vi "Lang Set Desc b.vi"(8 "error in (no error)":errorcluster, 10 "b":T1, 11 "LF2R IDE in":refnum<class "Main Panel.lvclass">) -> (0 "error out":errorcluster, 3 "LF2R IDE out":refnum<class "Main Panel.lvclass">)   [LabVIEW 2018, in "Framework.lvlib" / "Framework.lvclass"]
uses:
  Framework/Framework/Framework.lvclass
  Main Panel.lvclass
  D:/project/hobby/LabVIEW/LF2R/LabVIEW/Source/Actor/Framework/Framework/Framework.lvclass
  C:/Program Files (x86)/National Instruments/LabVIEW 2018/vi.lib/MGI/Panel Manager/Panel Actor/Panel Actor/Panel Actor.lvclass
  C:/Program Files (x86)/National Instruments/LabVIEW 2018/vi.lib/MGI/Monitored Actor/Monitored Actor/Monitored Actor/Monitored Actor.lvclass
  C:/Program Files (x86)/National Instruments/LabVIEW 2018/vi.lib/ActorFramework/Actor/Actor.lvclass
  Const Lang Property.ctl
  Const UI Desc Frame b.ctl
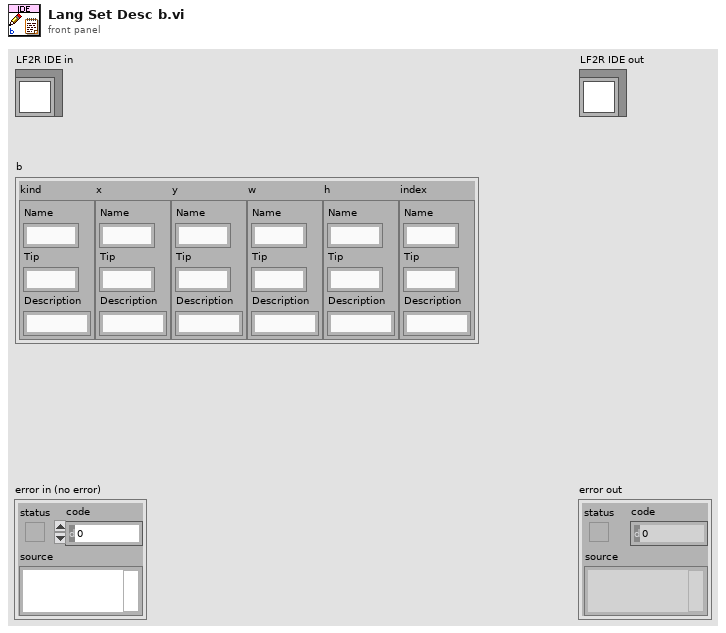
[diagram p1: front panel]
types:
  T1 = typedef "Framework.lvlib/Framework.lvclass/Const UI Desc Frame b.ctl" = cluster{"kind":T2, "x":T2, "y":T2, "w":T2, "h":T2, "index":T2}
  T2 = typedef "Framework.lvlib/Framework.lvclass/Const Lang Property.ctl" = cluster{"Name":string, "Tip":string, "Description":string}
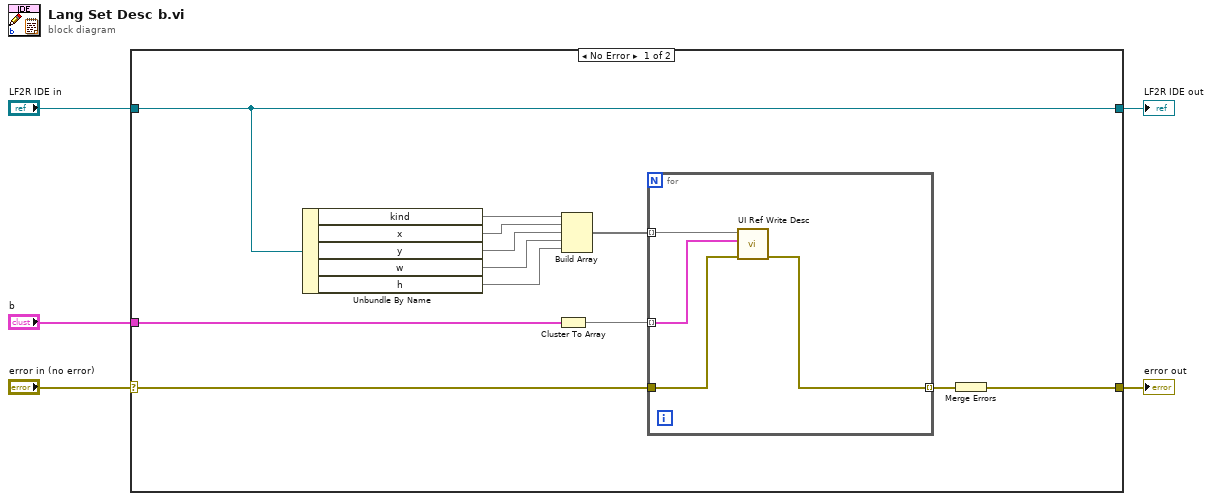
[diagram p0: block diagram]
diagram:
  n1 = case shown="No Error" "error in (no error)" {
    selector: "error in (no error)" -> [w13 w23]
    tunnel: [w11 w23] -> w4
    tunnel: [w17 w22] -> w2
    tunnel: "LF2R IDE in" -> [w17 w22]
    tunnel: "b" -> [w15 _]
    frame No Error {
      n2 = Unbundle By Name(w17) -> ("kind"=w10, "x"=w9, "y"=w8, "w"=w7, "h"=w6)
      n3 = Cluster To Array(cluster=w15) -> (array=w14:T2[])
      n4 = Build Array(w10, w9, w8, w7, w6) -> (w16:void[])
      n5 = for {
        tunnel: w16 -> [w18] mode=indexing
        tunnel: w14 -> [w21] mode=indexing
        tunnel: w13 -> [w20]
        tunnel: [w19] -> w12 mode=indexing
        n6 = call "UI Ref Write Desc.vi"("error in (no error)"=w20, "UI Property"=w21, "UI Ref"=w18) -> ("error out"=w19:errorcluster)  [unwired: 8 in]
      }
      n7 = Merge Errors(w12) -> (w11:errorcluster)
    }
    frame Error {
    }
  }
  "error out" <- w4
  "LF2R IDE out" <- w2
